vi "Indices to Set.vi"(8 "error in (no error)":errorcluster, 11 "Index Types":T1[](array[typedef])) -> (0 "error out":errorcluster, 3 "Index Type Set":T3)   [LabVIEW 2020, in "Current Value Table(Rebuild).lvlib"]
uses:
  Type Defs/Typed Index Set.ctl
  Type Defs/Data Types.ctl
  Type Defs/Index Types.ctl
  Errors/Generate Error.vi
  Current Value Table(Rebuild).lvlib
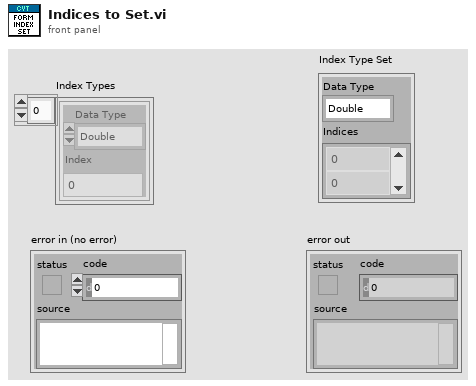
[diagram p1: front panel]
types:
  T1 = typedef "Current Value Table(Rebuild).lvlib/Index Types.ctl" = cluster{"Data Type":T2, "Index":i32}
  T2 = typedef "Current Value Table(Rebuild).lvlib/Data Types.ctl" = enum16{"Double", "Single", "I64", "I32", "I16", "I8", "U64", "U32", "U16", "U8", "String", "Boolean", "Array of U8", "Array of U16", "Array of U32", "Array of U64", "Array of I64", "Array of I32", "Array of I16", "Array of I8", "Array of Double", "Array of Single", "Array of Boolean", "Array of String"}
  T3 = typedef "Current Value Table(Rebuild).lvlib/Typed Index Set.ctl" = cluster{"Data Type":T2, "Indices":i32[]}
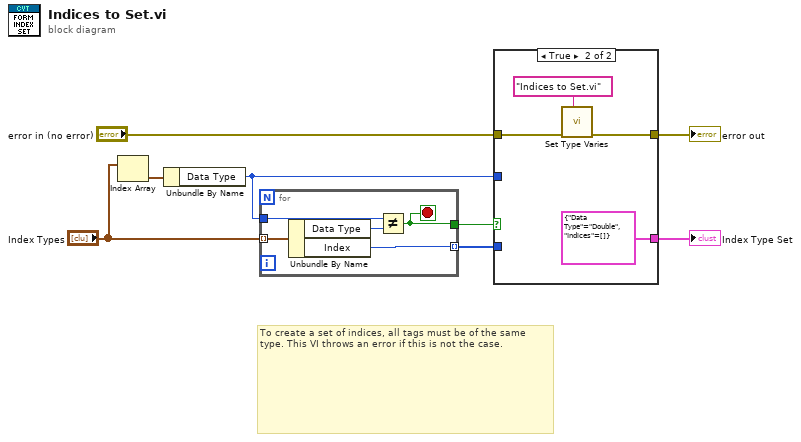
[diagram p0: block diagram]
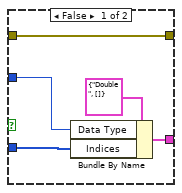
[diagram p2: hidden frame]
diagram:
  # "To create a set of indices, all tags must be of the same type. This VI throws an error if this is not the case."
  n1 = Index Array(array="Index Types") -> (element=w7:T1)  [unwired: 1 in]
  n2 = Unbundle By Name(w7) -> ("Data Type"=w4:T2)
  n3 = for {
    tunnel: "Index Types" -> [w13] mode=indexing
    tunnel: w4 -> [w10]
    tunnel: [w12] -> w5 mode=indexing
    tunnel: [w11] -> w6
    stop <- w11 stop-if-true
    n4 = Unbundle By Name(w13) -> ("Data Type"=w9:T2, "Index"=w12:i32)
    n5 = Not Equal?(x=w10, y=w9) -> (x != y?=w11:bool)
  }
  n6 = case shown="True" w6 {
    tunnel: w5 -> [w16 _]
    tunnel: w4 -> [w17 _]
    tunnel: [w15 T3 {"Data Type"=enum."Double", "Indices"=[]} ("Index Type Set")] -> w3
    tunnel: "error in (no error)" -> [w14 w21]
    tunnel: [w14 w20] -> w1
    frame False {
      n7 = Bundle By Name(cluster=T3 {"Data Type"=enum."Double", "Indices"=[]} ("Index Type Set"), "Data Type"=w17, "Indices"=w16) -> (w15:T3)
    }
    frame True {
      n8 = call "Set Type Varies.vi"("caller name"="Indices to Set.vi", "error in (no error)"=w21) -> ("error out"=w20:errorcluster)  [unwired: 9 in]
    }
  }
  "Index Type Set" <- w3
  "error out" <- w1
